vi "LIA_FPGA-Experimental.vi"() -> (1 "K Constant":fxp<+/-,32,16>, 2 "Nominal Freq":fxp<+/-,64,32>)   [LabVIEW 2012]
uses:
  <vilib>/rvi/DataTransferAndStorage/Container/Common/niFpgaContainerMetaDataKey.ctl
  <vilib>/rvi/DataTransferAndStorage/Container/Common/niFpgaContainerState.ctl
  <vilib>/rvi/DataTransferAndStorage/Container/Common/niFpgaDataTypeControl.ctl
  <vilib>/rvi/DataTransferAndStorage/Container/Common/niFpgaContainerImplementationControl.ctl
  <vilib>/rvi/DataTransferAndStorage/Container/Common/niFpgaContainerArbitrationOptionsControl.ctl
  <vilib>/rvi/DataTransferAndStorage/Container/Common/niFpgaTransferTypeControl.ctl
  <vilib>/rvi/DataTransferAndStorage/Container/Common/niFpgaContainerInitializationParameters.ctl
  <vilib>/rvi/Memory/Memory_Types/niFpgaMemoryInterfaceConfiguration.ctl
  <vilib>/rvi/FIFO/Fifo_Types/niFpgaFifoControlLogicControl.ctl
  <vilib>/rvi/FXPMathLib/FxpSinAndCos/subVIs/nifxpmath_SinAndCos_SimConfig.ctl
  <vilib>/rvi/FXPMathLib/basic elements/FxpIntAccumulator/subVIs/nifxpmath_IntAccumulator_SimConfig.ctl
  <vilib>/Platform/TimedLoop/XDataNode/timing_clust.ctl
  <vilib>/Platform/TimedLoop/XDataNode/nitl_modes.ctl
  <vilib>/Platform/TimedLoop/XDataNode/wakeup.ctl
  <vilib>/rvi/DataTransferAndStorage/Container/Common/niFpgaContainerGetUniqueNameForEmu.vi
  <vilib>/rvi/DataTransferAndStorage/Container/Common/niFpgaContainerSetEmuInfo.vi
  <vilib>/rvi/eio/common/nirviEmuReportErrorAndStop.vi
  <vilib>/rvi/eio/common/nirviEmuTemplateMethod_errors.vi
  <vilib>/rvi/interface/RandomDataEmulation/nirviRandomDataFPGAFIFO.vi
  <vilib>/rvi/interface/RandomDataEmulation/niFpgaRandomDataHandleErrors.vi
  <vilib>/rvi/FXPMathLib/FxpSinAndCos/simVIs/DllFxpSinAndCosTemp_sub.vi
  <vilib>/rvi/FXPMathLib/basic elements/FxpIntAccumulator/simVIs/DllFxpIntAccumulator_sub.vi
  <vilib>/rvi/Emulation/niFpgaSctlEmulationGetInTimedLoop.vi
  <vilib>/rvi/FIFO/Fifo_Resource/nirvififoEmulationSetSize.vi
  <vilib>/rvi/errors/niFpgaSetErrorForExecOnDevCompSimple.vi
  <vilib>/rvi/Emulation/niFpgaSctlEmulationFifoFullMgr.vi
  <vilib>/rvi/Emulation/niFpgaSctlEmulationResourceMgr.vi
  <vilib>/rvi/Emulation/niFpgaSctlEmulationRegisterWithScheduler.vi
  <vilib>/rvi/Emulation/niFpgaSctlEmulationScheduler.vi
  <vilib>/rvi/LocalResourceManager/LocalResourceManager.xnode
  <vilib>/eio/EIONode/EIONode.xnode
  <vilib>/rvi/DataTransferAndStorage/Container/XNode/niFpgaContainer.xnode
  <vilib>/rvi/interface/RandomDataEmulation/nirviRandomDataFpgaReadWriteTemplate.vi
  <vilib>/rvi/FXPMathLib/FxpSinAndCos/XNode/nifxpmath_SinAndCos.xnode
  <vilib>/rvi/FXPMathLib/basic elements/FxpIntAccumulator/XNode/nifxpmath_IntAccumulator.xnode
  <vilib>/Platform/TimedLoop/XDataNode/XDataNode.xnode
  <vilib>/rvi/FXPMathLib/FxpInterpret/XNode/nifxpmath_Interpret.xnode
  <vilib>/rvi/FIFO/Fifo_Resource/nirvififoEmulationWrite.vi
  <vilib>/rvi/FIFO/Fifo_Resource/nirvififoEmulationRead.vi
  <vilib>/Platform/TimedLoop/XDataNode/XDNodeRunTimeDep.lvlib
panel:
  in  "Nominal Frequency":fxp<+/-,64,32>
  in  "VCO Constant":fxp<+/-,64,10>
  in  "PID Error":fxp<+/-,64,32>
  in  "Case Number":i16
  in  "DAQ Acquisition Rate":i16
  out "Ticks":i16
  out "TF Input":fxp<+/-,64,32>
  out "Sine Output":fxp<+/-,64,32>
  out "Numeric":fxp<+/-,64,32>
  in  "Voltage (V)":fxp<+,64,12>=3276.8125
  out "Summation":fxp<+/-,64,32>
  out "Corrected Frequency":fxp<+/-,64,32>
  out "Angular Frequency":fxp<+/-,64,32>
  out "Z":fxp<+/-,64,32>
  in  "Start":bool
  out "Radians":fxp<+/-,14,5>
  out "Cos":fxp<+/-,14,2>
  out "Sin":fxp<+/-,14,2>
  in  "Period":u16=1000
  out "ticks":u32
  out "ref":i16 format="%.0x"
  out "sig":i16 format="%.0x"
  out "channelQ":i64
  out "channelI":i64
  out "f":fxp<+/-,32,0> format="%.32g"
  in  "dec2":i16=1
  in  "K":fxp<+,16,0>=0.001007080078125
  in  "nominal freq":fxp<+,16,0>=0.010009765625
  in  "dec1":i16=1
  in  "stages":i8=1
  in  "stop":bool
  in  "decimation":i16=1024
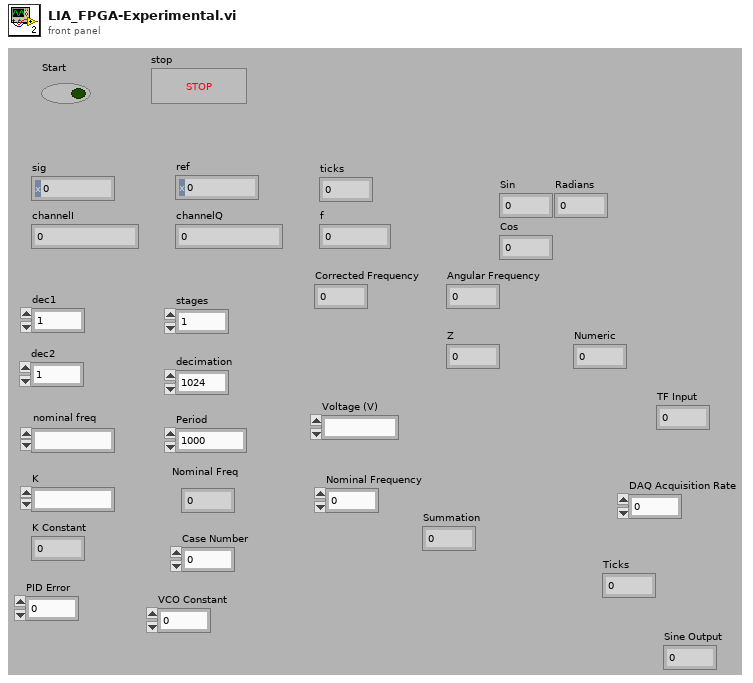
[diagram p1: front panel]
types:
  T1 = typedef "XDNodeRunTimeDep.lvlib/timing_clust.ctl" = cluster{"Expected End [f-1]":u64, "Actual End [f-1]":u64, "Finished Late? [f-1]":bool, "Expected End [i-1]":u64, "Actual End [i-1]":u64, "Finished Late? [i-1]":bool, "Expected Start [i]":u64, "Actual Start [i]":u64, "Expected Start [f]":u64, "Actual Start [f]":u64, "Source Name":string, "Structure Name":string, "Period":i64, "Deadline":i64, "Offset":i64, "Start":i64, "Priority":i32, "Timeout":i32, "Mode":T2, "Wakeup Reason":T3, "Error":errorcluster, "Source Type":string, "Secondary Source Type":string, "Global End Time":u64, "Global Start Time":u64, "Frame Duration":u64, "Iteration Duration":u64, "Assigned CPU":i32, "I/O Scan Engine Mode":u32}
  T2 = typedef "XDNodeRunTimeDep.lvlib/nitl_modes.ctl" = enum32{"No Change", "Process missed periods, maintain original phase", "Discard missed periods, maintain original phase", "Process missed periods, ignore original phase", "Discard missed periods, ignore original phase"}
  T3 = typedef "XDNodeRunTimeDep.lvlib/wakeup.ctl" = enum32{"Normal", "Aborted", "Asynchronous wakeup", "Timing source error", "Timed loop error", "Timeout"}
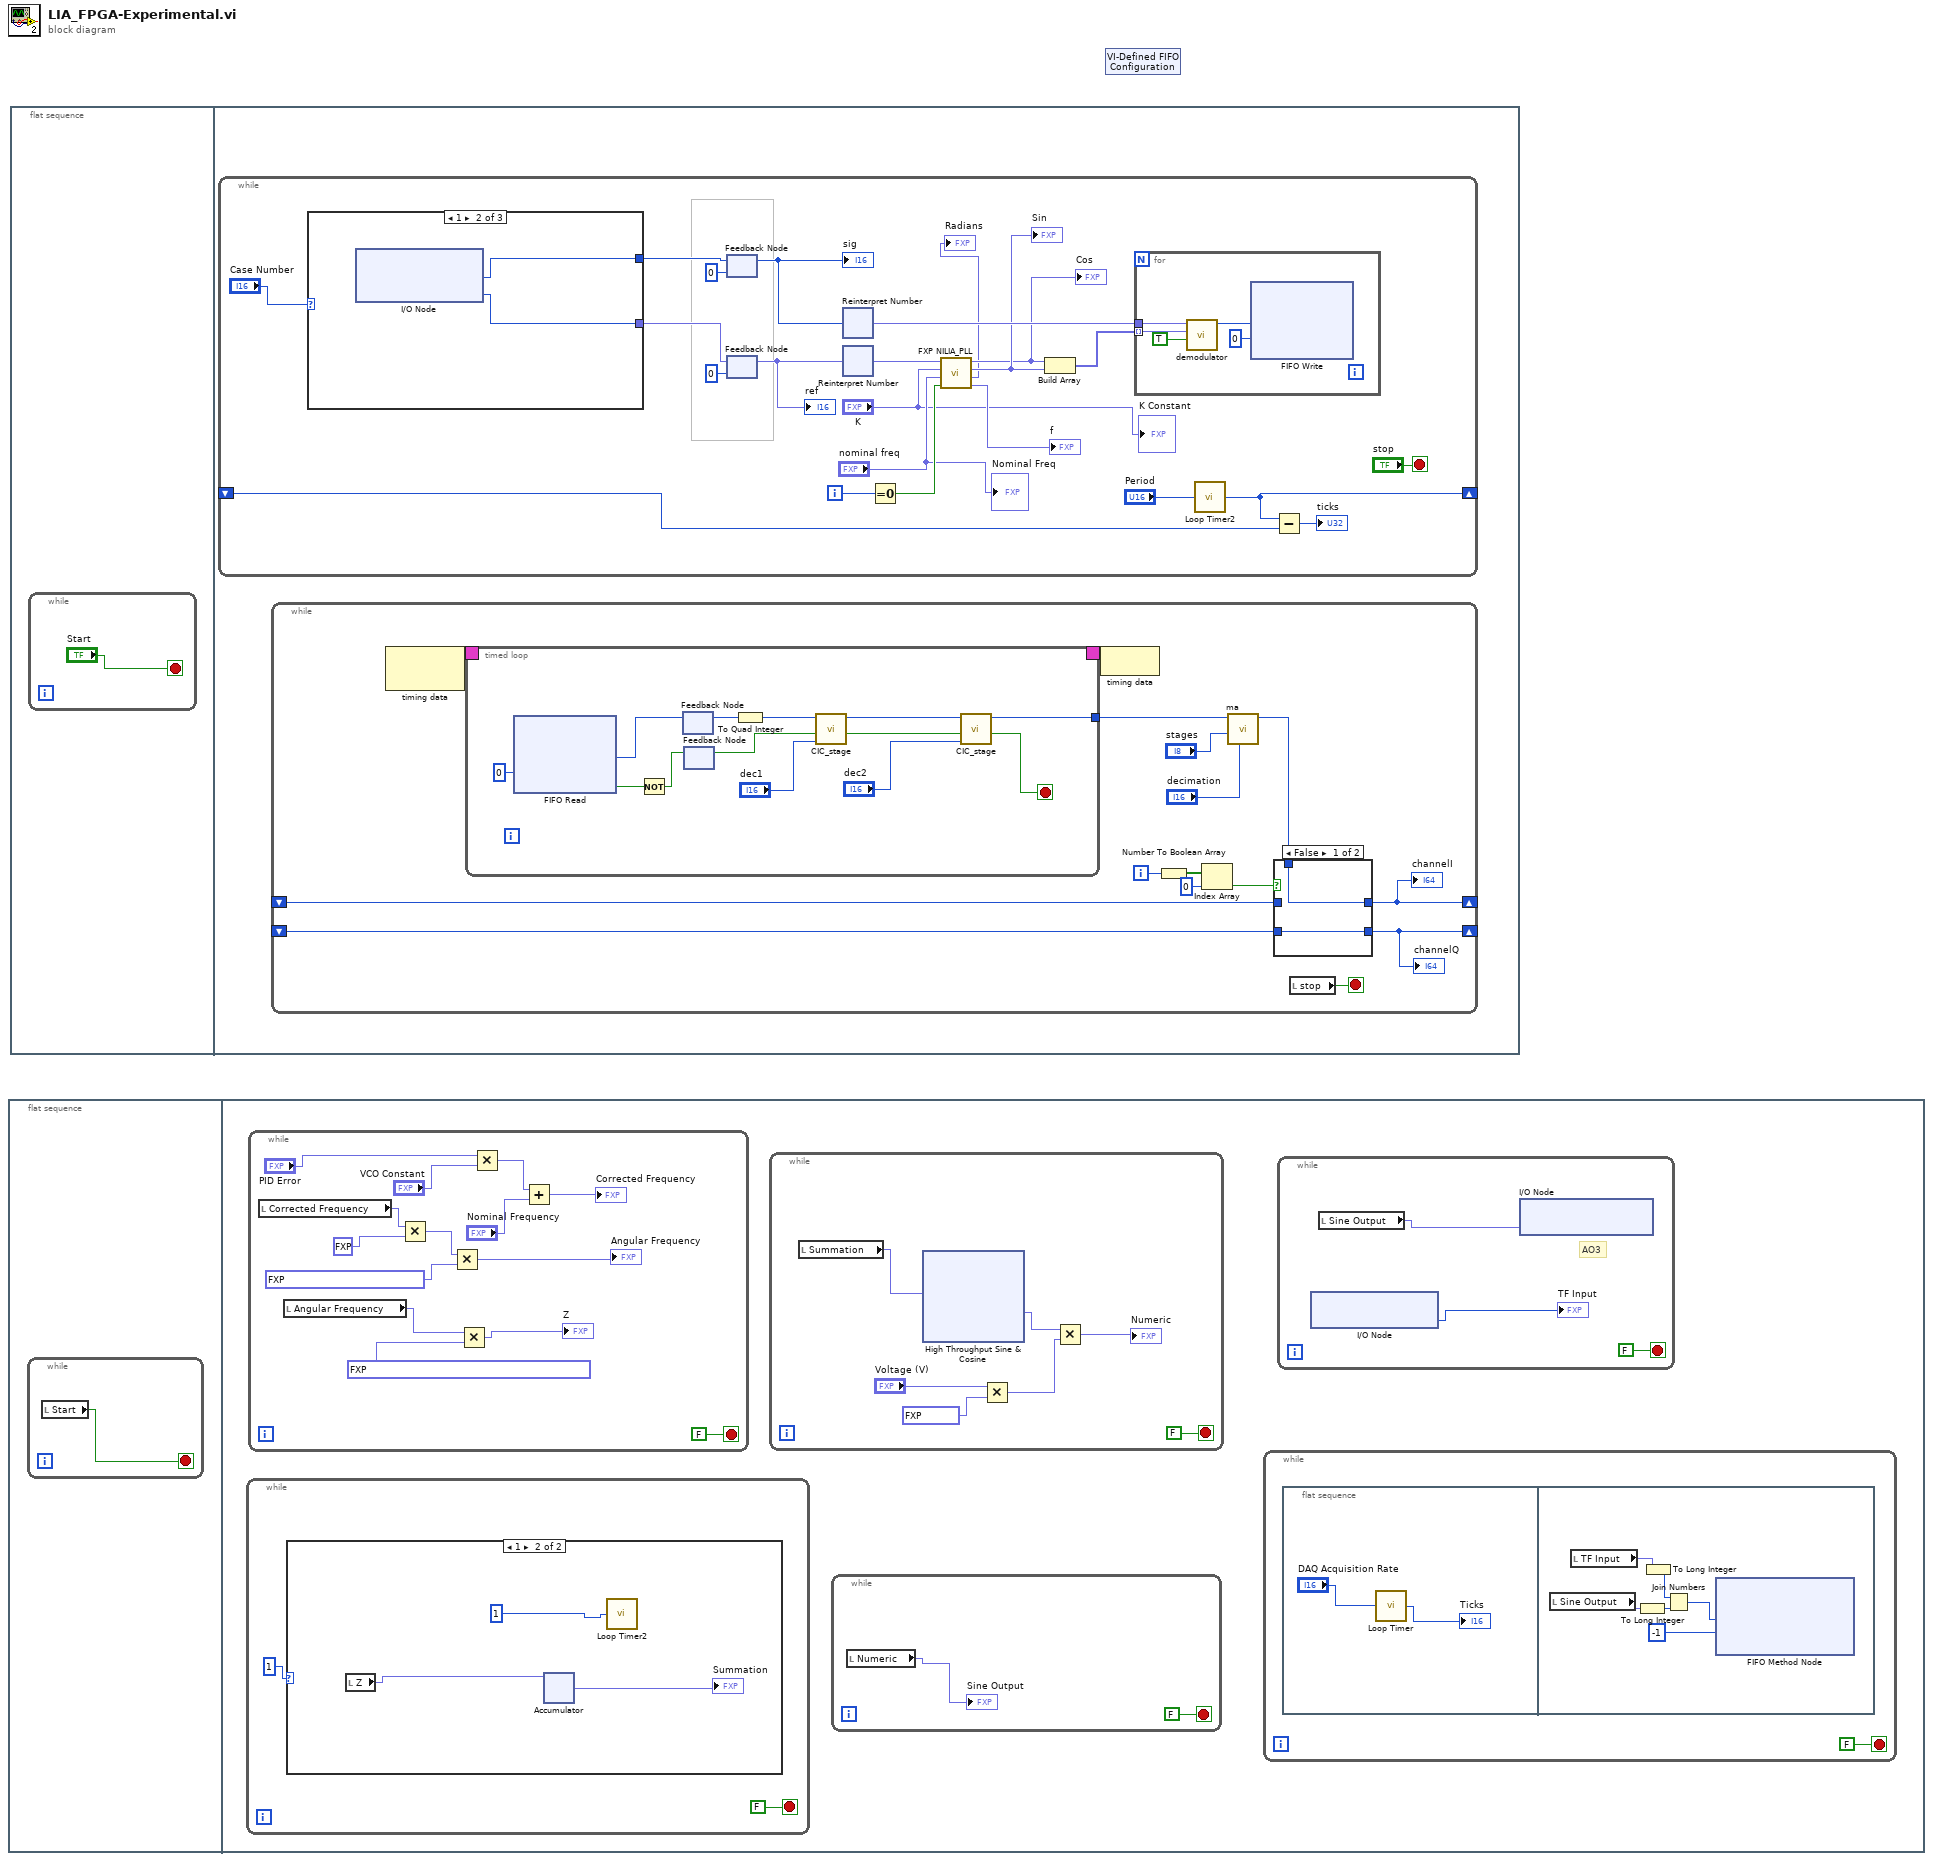
[diagram p0: block diagram]
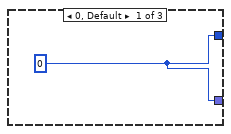
[diagram p3: hidden frame]
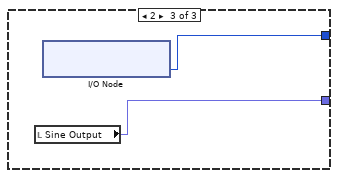
[diagram p4: hidden frame]
diagram:
  n1 = flat-sequence {
    frame #0 {
      n2 = while {
        stop <- w1 stop-if-true
        n3 = local read "Start"() -> (w1:bool)
      }
    }
    frame #1 {
      n4 = while {
        stop <- FALSE stop-if-true
        n5 = case shown="1" 1 {
          frame 0, Default {
          }
          frame 1 {
            n6 = local read "Z"() -> (w57:fxp<+/-,64,32>)
            n7 = xnode "Accumulator"("x"=w57) -> ("s"=→"Summation":fxp<+/-,64,32>)  [unwired: 4 in, 1 out]
            n8 = call "Loop Timer2"("Count(uSec)"=1) -> ()  [unwired: 1 out]
          }
        }
      }
      n9 = while {
        stop <- FALSE stop-if-true
        n10 = local read "Corrected Frequency"() -> (w90:fxp<+/-,64,32>)
        n11 = local read "Angular Frequency"() -> (w95:fxp<+/-,64,32>)
        n12 = Multiply(x=w90, y=fxp<+,1,2> 2.0) -> (x*y=w93:fxp<+/-,64,33>)
        n13 = Multiply(x=w93, y=fxp<+,30,2> 3.1415926814079285) -> (x*y=→"Angular Frequency":fxp<+/-,64,35>)
        n14 = Multiply(x=w95, y=fxp<+,46,7> 0.0010000000002037268) -> (x*y=→"Z":fxp<+/-,64,39>)
        n15 = Multiply(x="PID Error", y="VCO Constant") -> (x*y=w87:fxp<+/-,64,42>)
        n16 = Add(x=w87, y="Nominal Frequency") -> (x+y=→"Corrected Frequency":fxp<+/-,64,43>)
      }
      n17 = while {
        stop <- FALSE stop-if-true
        n18 = local read "Summation"() -> (w21:fxp<+/-,64,32>)
        n19 = xnode "High Throughput Sine & Cosine"("x (pi)"=w21) -> ("sin(x)"=w20:fxp<+/-,16,2>)  [unwired: 1 out]
        n20 = Multiply(x="Voltage (V)", y=fxp<+,17,12> 3276.8125) -> (x*y=w16:fxp<+,64,24>)
        n21 = Multiply(x=w20, y=w16) -> (x*y=→"Numeric":fxp<+/-,64,26>)
      }
      n22 = while {
        stop <- FALSE stop-if-true
        n23 = local read "Numeric"() -> (→"Sine Output":fxp<+/-,64,32>)
      }
      n24 = while {
        stop <- FALSE stop-if-true
        n25 = flat-sequence {
          frame #0 {
            n26 = call "Loop Timer"("Count(uSec)"="DAQ Acquisition Rate") -> ("Tick Count(uSec)"=→"Ticks":u32)
          }
          frame #1 {
            n27 = local read "Sine Output"() -> (w6:fxp<+/-,64,32>)
            n28 = local read "TF Input"() -> (w8:fxp<+/-,64,32>)
            n29 = To Long Integer(number=w6) -> (32bit integer=w7:i32)
            n30 = To Long Integer(number=w8) -> (32bit integer=w9:i32)
            n31 = Join Numbers(hi=w9, lo=w7) -> ((hi.lo)=w5:u64)
            n32 = xnode ("FIFO Method Node")("Element"=w5, "Timeout"=-1) -> ()  [unwired: 1 in, 2 out]
          }
        }
      }
      n33 = while {
        stop <- FALSE stop-if-true
        # "AO3"
        n34 = xnode "I/O Node"() -> ("Connector0/AI6"=→"TF Input":i16)  [unwired: 1 in, 1 out]
        n35 = local read "Sine Output"() -> (w12:fxp<+/-,64,32>)
        n36 = xnode "I/O Node"("Connector0/AO3"=w12) -> ()  [unwired: 1 in, 1 out]
      }
    }
  }
  n37 = flat-sequence {
    frame #0 {
      n38 = while {
        stop <- "Start" stop-if-true
      }
    }
    frame #1 {
      n39 = while {
        shift-right: [w119] -> _
        shift-left: _ -> [w118]
        i -> [w122]
        stop <- "stop" stop-if-true
        n40 = case shown="1" "Case Number" {
          tunnel: [w123 w125 w127] -> w101
          tunnel: [w123 w124 w126] -> w100
          frame 0, Default {
            w123 = 0
          }
          frame 1 {
            n41 = xnode "I/O Node"() -> ("Connector0/AI6"=w125:i16, "Connector0/AI7"=w124:i16)  [unwired: 2 in, 2 out]
          }
          frame 2 {
            n42 = local read "Sine Output"() -> (w126:fxp<+/-,64,32>)
            n43 = xnode "I/O Node"() -> ("Connector0/AI6"=w127:i16)  [unwired: 1 in, 1 out]
          }
        }
        n44 = feedback #1(i16 0 ("y")) -> (w112:i32)
        "sig" <- w112
        n45 = feedback-in #1(w101) -> ()
        n46 = feedback #2(i16 0 ("z [I32.1]")) -> (w111:fxp<+/-,64,32>)
        "ref" <- w111
        n47 = feedback-in #2(w100) -> ()
        n48 = xnode "Reinterpret Number"("x"=w112) -> ("y"=w115:fxp<+/-,32,1>)
        n49 = xnode "Reinterpret Number"("x"=w111) -> ("y"=w110:fxp<+/-,64,1>)
        n50 = Equal To 0?(x=w122) -> (x = 0?=w108:bool)
        n51 = call "FXP NILIA_PLL.vi"("reset?"=w108, "norminal freq [U16.0]"="nominal freq", "alpha [U16.0]"="K", "x[I16.1]"=w110) -> ("f"=→"f":fxp<+/-,32,0>, "z [I32.1]"=→"Radians":fxp<+/-,32,1>, "sin(z)"=w105:fxp<+/-,16,2>, "cos(z)"=w104:fxp<+/-,16,2>)  [unwired: 4 in]
        "Sin" <- w105
        "Cos" <- w104
        n52 = Build Array(w104, w105) -> (w116:fxp<+/-,16,2>[])
        n53 = for {
          tunnel: w115 -> [w130]
          tunnel: w116 -> [w128] mode=indexing
          n54 = call "demodulator.vi"("New Data"=TRUE, "ref"=w128, "signal"=w130) -> ("x*y"=w131:i32)  [unwired: 8 out]
          n55 = xnode ("FIFO Write")("Element"=w131, "Timeout"=0) -> ()  [unwired: 1 in, 2 out]
        }
        n56 = call "Loop Timer2"("Count(uSec)"="Period") -> ("Tick Count(uSec)"=w119:u32)
        n57 = Subtract(x=w119, y=w118) -> (x-y=→"ticks":u32)
        "Nominal Freq" <- "nominal freq"
        "K Constant" <- "K"
      }
      n58 = while {
        shift-right: [w134] -> _
        shift-left: _ -> [w136]
        shift-right: [w133] -> _
        shift-left: _ -> [w135]
        i -> [w141]
        stop <- w143 stop-if-true
        n59 = node-c288() -> (w147:T1)  [unwired: 1 out]
        n60 = timed-loop {
          timing: w147 -> [_]
          timing-out: [_] -> w146
          tunnel: [w155] -> w142
          stop <- w154 stop-if-true
          n61 = xnode ("FIFO Read")("Timeout"=0) -> ("Element"=w162:i32, "Timed Out?"=w161:bool)  [unwired: 1 in, 1 out]
          n62 = Not(x=w161) -> (.not. x?=w160:bool)
          n63 = feedback-in #3(w162) -> ()
          n64 = feedback #3() -> (w164:i32)  [unwired: 1 out]
          n65 = feedback-in #4(w160) -> ()
          n66 = feedback #4() -> (w158:bool)  [unwired: 1 out]
          n67 = To Quad Integer(1:w164) -> (0:w159:i64)
          n68 = call "CIC_stage.vi"("decimate factor"="dec1", "New Data"=w158, "input"=w159) -> ("Data Ready"=w156:bool, "output"=w157:i64)  [unwired: 7 out]
          n69 = call "CIC_stage.vi"("decimate factor"="dec2", "New Data"=w156, "input"=w157) -> ("Data Ready"=w154:bool, "output"=w155:i64)  [unwired: 7 out]
        }
        n70 = node-c288(w146) -> ()
        n71 = Number To Boolean Array(number=w141) -> (Boolean array=w140:bool[])
        n72 = Index Array "Index Array"(array=w140, index=0) -> (element=w138:bool)
        n73 = call "ma.vi"("decimate"="decimation", "stages"="stages", "input"=w142) -> ("output"=w137:i64)  [unwired: 8 out]
        n74 = case shown="False" w138 {
          tunnel: w137 -> [w149 w151]
          tunnel: [w149 w150] -> w134
          tunnel: [w148 w151] -> w133
          tunnel: w136 -> [_ w150]
          tunnel: w135 -> [w148 _]
          frame False {
          }
          frame True {
          }
        }
        "channelI" <- w134
        "channelQ" <- w133
        n75 = local read "stop"() -> (w143:bool)
      }
    }
  }
  n76 = xnode "VI-Defined FIFO Configuration"() -> ()  [unwired: 1 out]
